vi "Preconditioning.vi"(8 "error in (no error)":errorcluster, 10 "Sequence Context":refnum<k7>, 11 "PreUUT in":refnum<class "PreUUT.lvclass">) -> (0 "error out":errorcluster, 2 "Preconditioning":bool, 3 "PreUUT out":refnum<class "PreUUT.lvclass">)   [LabVIEW 2019, in "OPC UA.lvlib" / "PreUUT.lvclass"]
uses:
  PreUUT.lvclass
  C:/Workspace/battery-submodule-eol_oop/Sequence/CodeModules/OPC UA Client/OPC UA/OPC UA.lvclass
  OPC UA/OPC UA.lvclass/OPC UA.ctl
  <vilib>/addons/TestStand/_TSUtility.llb/TestStand - Get Property Value (String).vi
  <vilib>/addons/TestStand/_TSUtility.llb/TestStand - Set Property Value (String).vi
  <vilib>/addons/TestStand/_TSUtility.llb/TestStand - Set Property Value (Number {Signed 32-bit Integer}).vi
  OPC UA/OPC UA.lvclass
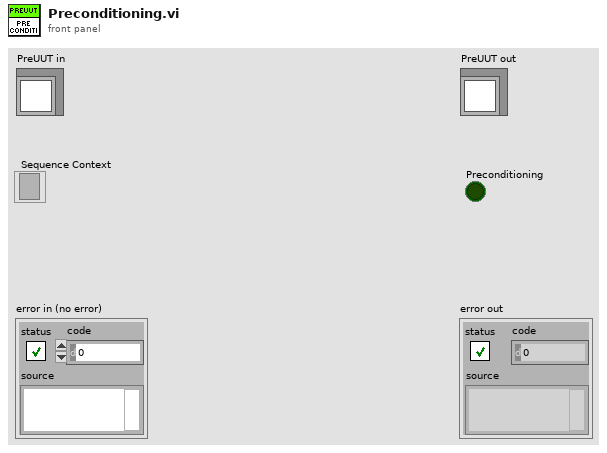
[diagram p1: front panel]
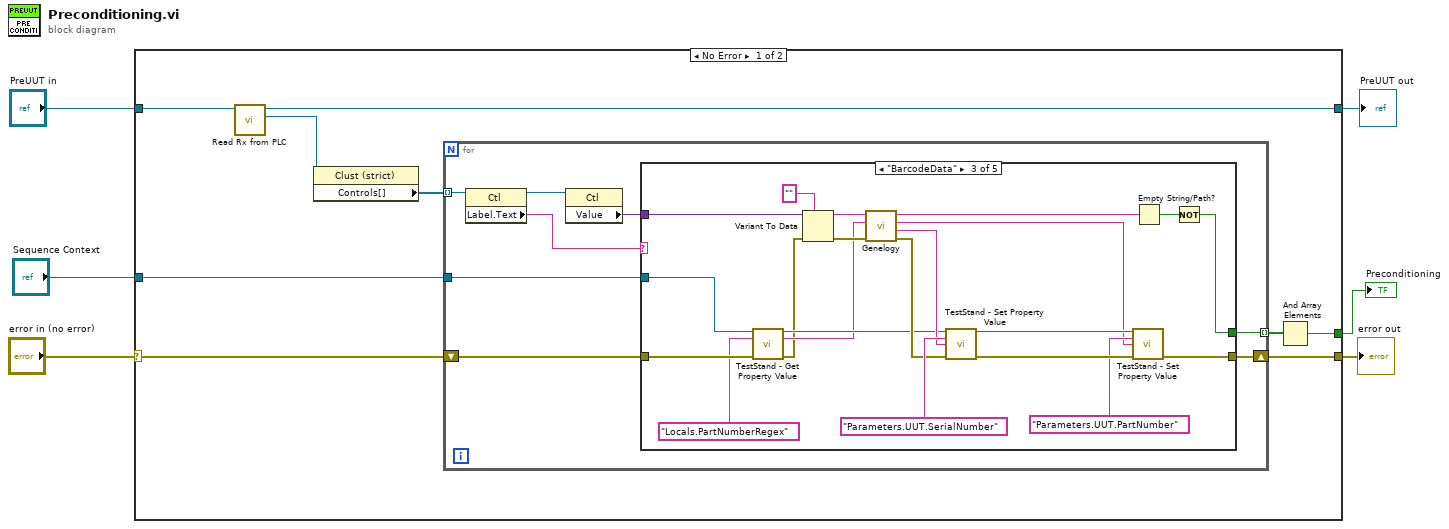
[diagram p0: block diagram]
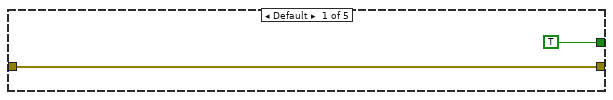
[diagram p2: hidden frame]
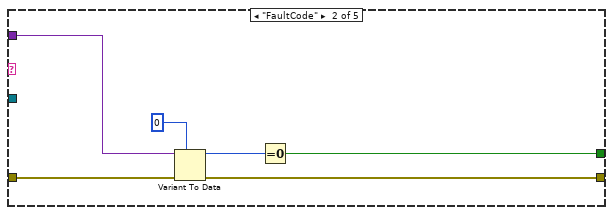
[diagram p3: hidden frame]
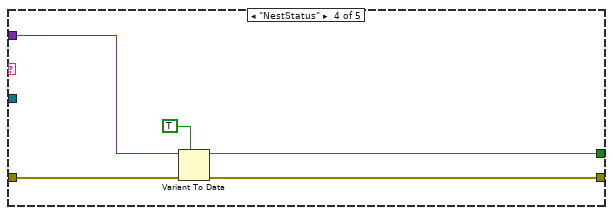
[diagram p4: hidden frame]
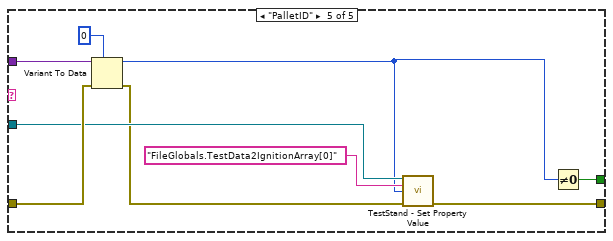
[diagram p5: hidden frame]
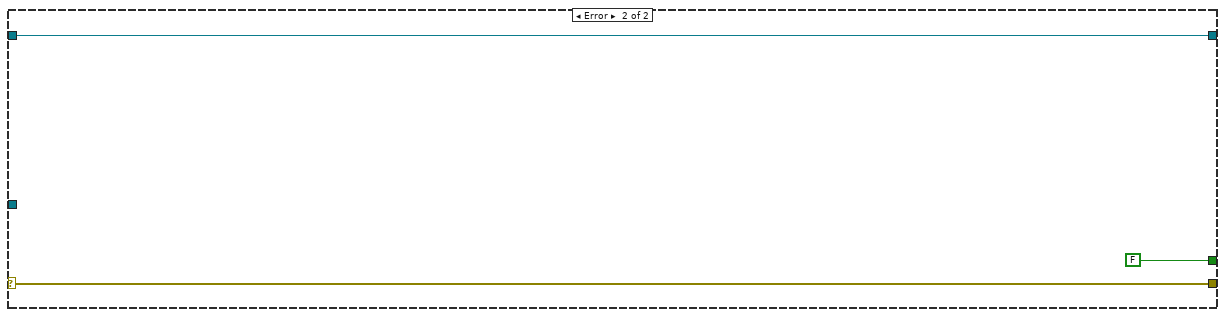
[diagram p6: hidden frame]
diagram:
  n1 = case shown="No Error" "error in (no error)" {
    selector: "error in (no error)" -> [w14 w69]
    tunnel: [w13 w69] -> w5
    tunnel: [w9 w68] -> w3
    tunnel: "PreUUT in" -> [w10 w68]
    tunnel: [w12 FALSE] -> w2
    tunnel: "Sequence Context" -> [w7 _]
    frame No Error {
      n2 = call "Read Rx from PLC.vi"("OPC UA in"=w10) -> ("Rx from PLC"=w8:refnum<vi>, "OPC UA out"=w9:refnum<class "PreUUT.lvclass">)  [unwired: 8 in, 1 out]
      n3 = property class="Clust (strict)"(reference=w8) -> ("Controls[]"=w11:refnum<vi>[])  [unwired: 1 in, 2 out]
      n4 = for {
        tunnel: w11 -> [w23] mode=indexing
        shift-right: [w18] -> w13
        shift-left: w14 -> [w19]
        tunnel: w7 -> [w17]
        tunnel: [w16] -> w15 mode=indexing
        n5 = property class="Ctl"(reference=w23) -> (reference out=w21:refnum<vi>, "Label.Text"=w22:string)  [unwired: 1 in, 1 out]
        n6 = property class="Ctl"(reference=w21) -> ("Value"=w20:variant)  [unwired: 1 in, 2 out]
        n7 = case shown="\"BarcodeData\"" w22 {
          tunnel: w20 -> [_ w30 w52 w55 w65]
          tunnel: [TRUE w26 w39 w54 w63] -> w16
          tunnel: w19 -> [w25 w31 w38 w56 w66]
          tunnel: [w25 w29 w48 w53 w59] -> w18
          tunnel: w17 -> [_ _ w37 _ w62]
          frame Default {
          }
          frame "FaultCode" {
            n8 = Variant To Data(error in=w31, type=0, Variant=w30) -> (data=w27:i32, error out=w29:errorcluster)
            n9 = Equal To 0?(x=w27) -> (x = 0?=w26:bool)
          }
          frame "BarcodeData" {
            n10 = call-poly <vilib>:"TestStand - Get Property Value.vi"("Sequence Context In"=w37, "Lookup String"="Locals.PartNumberRegex", "error in (no error)"=w38) -> ("Sequence Context Out"=w36:refnum<k7>, "Value"=w33:string, "error out"=w32:errorcluster)  [unwired: 10 in]
            n11 = Variant To Data(error in=w32, type="", Variant=w52) -> (data=w34:string, error out=w46:errorcluster)
            n12 = call "Genelogy.vi"("error in"=w46, "PNSN Regex"=w33, "Barcode"=w34) -> ("error out"=w44:errorcluster, "SerialNumber"=w43:string, "PartNumber"=w42:string, "Revision"=w41:string)  [unwired: 5 in]
            n13 = call-poly <vilib>:"TestStand - Set Property Value.vi"("Sequence Context In"=w36, "Lookup String"="Parameters.UUT.SerialNumber", "New Value"=w43, "error in (no error)"=w44) -> ("Sequence Context Out"=w45:refnum<k7>, "error out"=w49:errorcluster)  [unwired: 10 in]
            n14 = call-poly <vilib>:"TestStand - Set Property Value.vi"("Sequence Context In"=w45, "Lookup String"="Parameters.UUT.PartNumber", "New Value"=w42, "error in (no error)"=w49) -> ("error out"=w48:errorcluster)  [unwired: 10 in, 1 out]
            n15 = Empty String/Path?(string/path=w41) -> (empty?=w40:bool)
            n16 = Not(x=w40) -> (.not. x?=w39:bool)
          }
          frame "NestStatus" {
            n17 = Variant To Data(error in=w56, type=TRUE, Variant=w55) -> (data=w54:bool, error out=w53:errorcluster)
          }
          frame "PalletID" {
            n18 = Variant To Data(error in=w66, type=0, Variant=w65) -> (data=w58:i32, error out=w60:errorcluster)
            n19 = call-poly <vilib>:"TestStand - Set Property Value.vi"("Sequence Context In"=w62, "Lookup String"="FileGlobals.TestData2IgnitionArray[0]", "New Value"=w58, "error in (no error)"=w60) -> ("error out"=w59:errorcluster)  [unwired: 10 in, 1 out]
            n20 = Not Equal To 0?(x=w58) -> (x != 0?=w63:bool)
          }
        }
      }
      n21 = And Array Elements(Boolean array=w15) -> (logical AND=w12:bool)
    }
    frame Error {
    }
  }
  "error out" <- w5
  "PreUUT out" <- w3
  "Preconditioning" <- w2
